vi "Add Header.vi"(8 "error in":errorcluster, 9 "value":string, 10 "header":T1, 11 "session in":refnum<class "Session.lvclass">) -> (0 "error out":errorcluster, 3 "session out":refnum<class "Session.lvclass">)   [LabVIEW 2019, in "NI_Advanced HTTP Client.lvlib" / "Session.lvclass"]
doc: "Adds a header field line to future web requests associated with the HTTP session. Headers define attributes of the data exchanged between the client and server."
uses:
  Session.lvclass
  Header--Combo Box.ctl
  Session.lvclass/Session.ctl
  lvwebclient_64.dll
  lvwebclient_32.dll
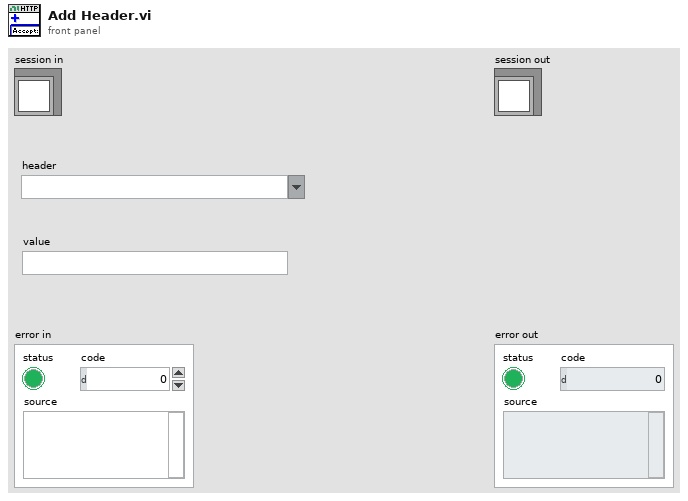
[diagram p1: front panel]
types:
  T1 = typedef "NI_Advanced HTTP Client.lvlib/Session.lvclass/Header--Combo Box.ctl" = string
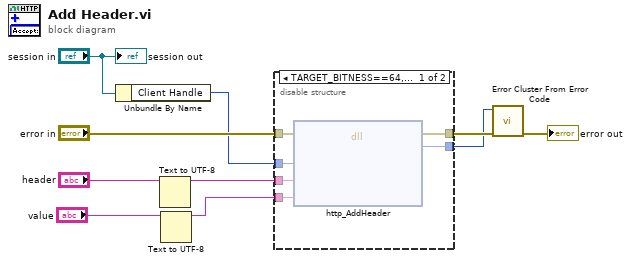
[diagram p0: block diagram]
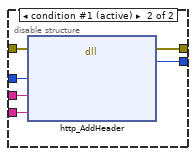
[diagram p2: hidden frame]
diagram:
  n1 = Unbundle By Name("session in") -> ("Client Handle"=w5:u32)
  n2 = Text to UTF-8(11:"header") -> (3:w3:string)  [unwired: 2 in, 1 out]
  n3 = Text to UTF-8(11:"value") -> (3:w1:string)  [unwired: 2 in, 1 out]
  n4 = disable-structure shown="TARGET_BITNESS==64, Default" {
    disable-tunnel: "error in" -> [w16 w22]
    disable-tunnel: [w15 w21] -> w7
    disable-tunnel: [w14 w20] -> w6
    disable-tunnel: w5 -> [w13 w19]
    disable-tunnel: w3 -> [w12 w18]
    disable-tunnel: w1 -> [w11 w17]
    frame condition #0 {
      n5 = dll-call lib="C:/Users/Localization Tester/Desktop/Advanced HTTP Client/lvwebclient_64.dll" fn="http_AddHeader"(error in=w16, "handle"=w13, "headerName"=w12, "headerValue"=w11) -> (error out=w15:errorcluster, "return"=w14:i32)  [unwired: 5 in, 1 out]
    }
    frame condition #1 (active) {
      n6 = dll-call lib="C:/Users/Localization Tester/Desktop/Advanced HTTP Client/lvwebclient_32.dll" fn="http_AddHeader"(error in=w22, "handle"=w19, "headerName"=w18, "headerValue"=w17) -> (error out=w21:errorcluster, "return"=w20:i32)  [unwired: 5 in, 1 out]
    }
  }
  n7 = call <vilib>:"Error Cluster From Error Code.vi"("error in (no error)"=w7, "error code (0)"=w6) -> ("error out"=→"error out":errorcluster)  [unwired: 7 in]
  "session out" <- "session in"
